vi "Device_Read.vi"(9 "queue out":refnum<queue>, 10 "Selected Count":i32, 11 "Device Handler pointer":i64[](array[numeric])) -> ()   [LabVIEW 2026]
uses:
  <vilib>/Platform/TimedLoop/XDataNode/timing_clust.ctl
  <vilib>/Platform/TimedLoop/XDataNode/nitl_modes.ctl
  <vilib>/Platform/TimedLoop/XDataNode/wakeup.ctl
  <vilib>/platform/TimedLoop/XDataNode/XDataNode.xnode
  <vilib>/Platform/TimedLoop/XDataNode/XDNodeRunTimeDep.lvlib
panel:
  in  "dataextraction":bool
  out "timed out? 3":bool
  out "concatenated string":string
  out "# elements in queue":i32
  out "element":u8[](array[numeric])
  out "timed out? 2":bool
  out "RX Return Value  2":i32
  out "CAN_Frame":u8[](array[numeric])
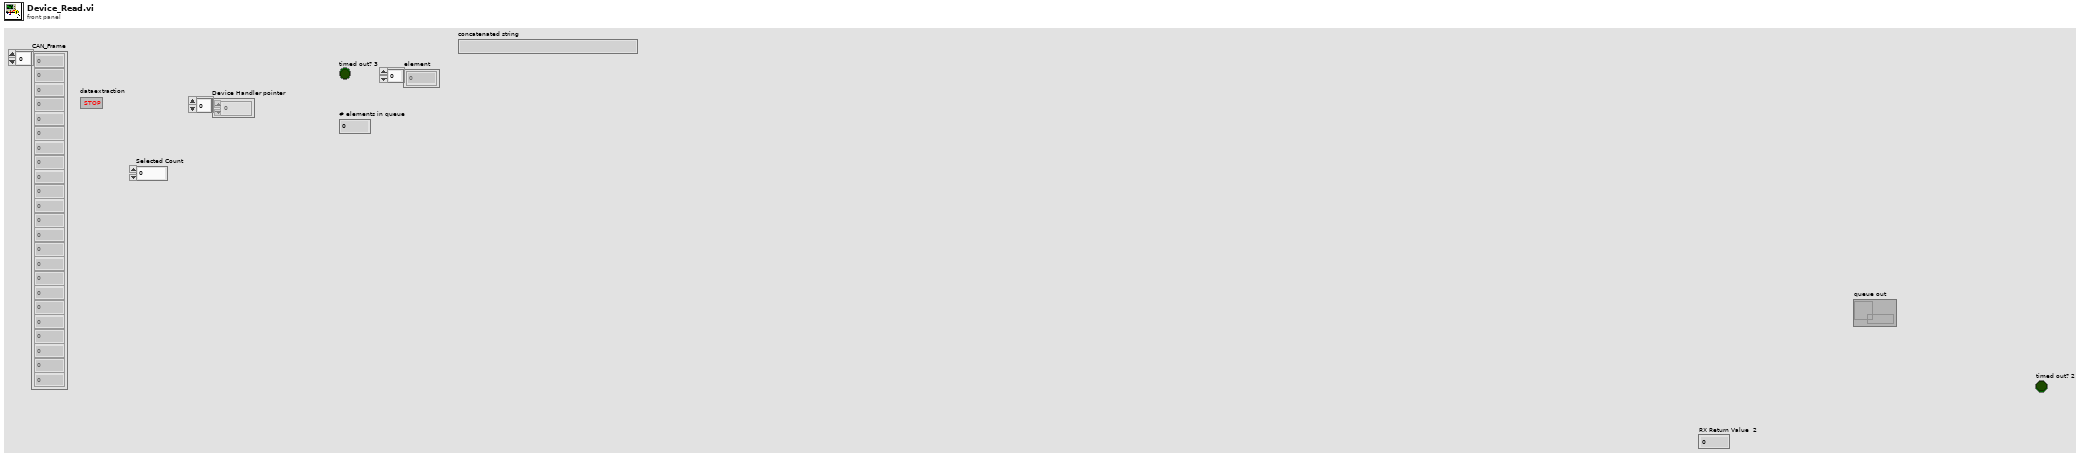
[diagram p1: front panel]
types:
  T1 = typedef "XDNodeRunTimeDep.lvlib/timing_clust.ctl" = cluster{"Expected End [f-1]":u64, "Actual End [f-1]":u64, "Finished Late? [f-1]":bool, "Expected End [i-1]":u64, "Actual End [i-1]":u64, "Finished Late? [i-1]":bool, "Expected Start [i]":u64, "Actual Start [i]":u64, "Expected Start [f]":u64, "Actual Start [f]":u64, "Source Name":string, "Structure Name":string, "Period":i64, "Deadline":i64, "Offset":i64, "Start":i64, "Priority":i32, "Timeout":i32, "Mode":T2, "Wakeup Reason":T3, "Error":errorcluster, "Source Type":string, "Secondary Source Type":string, "Global End Time":u64, "Global Start Time":u64, "Frame Duration":u64, "Iteration Duration":u64, "Assigned CPU":i32, "I/O Scan Engine Mode":u32}
  T2 = typedef "XDNodeRunTimeDep.lvlib/nitl_modes.ctl" = enum32{"No Change", "Process missed periods, maintain original phase", "Discard missed periods, maintain original phase", "Process missed periods, ignore original phase", "Discard missed periods, ignore original phase"}
  T3 = typedef "XDNodeRunTimeDep.lvlib/wakeup.ctl" = enum32{"Normal", "Aborted", "Asynchronous wakeup", "Timing source error", "Timed loop error", "Timeout"}
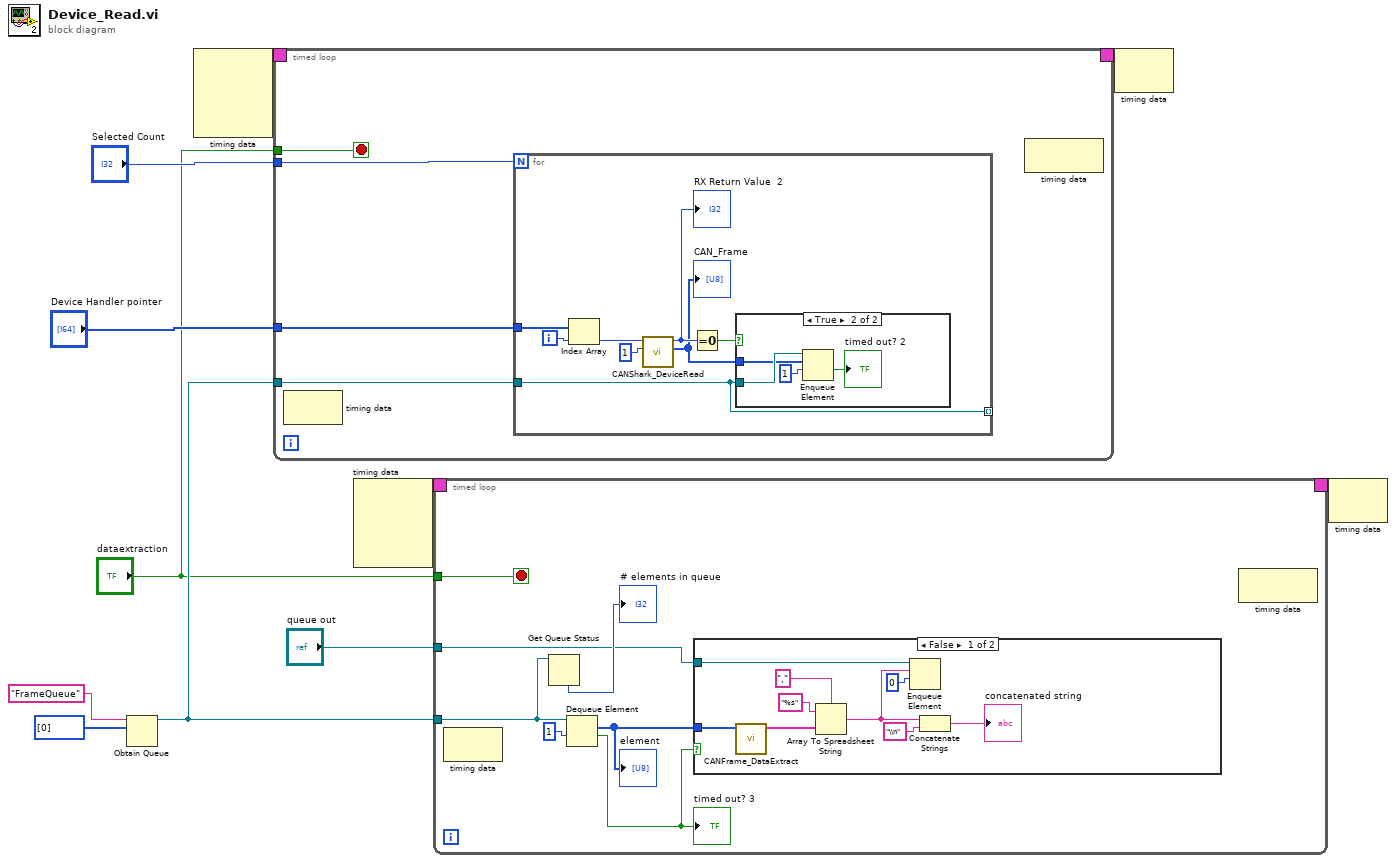
[diagram p0: block diagram]
diagram:
  n1 = Obtain Queue(name (unnamed)="FrameQueue", element data type=u8[] [0]) -> (queue out=w3:refnum<queue>)  [unwired: 3 in, 2 out]
  n2 = node-c288() -> (w11:T1)  [unwired: 4 in]
  n3 = timed-loop {
    timing: w11 -> [_]
    timing-out: [_] -> w10
    tunnel: "Device Handler pointer" -> [w15]
    tunnel: w3 -> [w14]
    tunnel: "Selected Count" -> [w13]
    tunnel: "dataextraction" -> [w12]
    stop <- w12 stop-if-true
    n4 = node-c288() -> ()  [unwired: 1 in, 1 out]
    n5 = for {
      N: w13 -> [_]
      tunnel: w15 -> [w21]
      tunnel: [w20] -> _ mode=indexing
      tunnel: w14 -> [w20]
      i -> [w22]
      n6 = Index Array(array=w21, index=w22) -> (element=w19:i64)
      n7 = call "CANShark_DeviceRead.vi"("Timeout"=1, "Device Handler"=w19) -> ("CAN_Frame"=w16:u8[], "RX Return Value"=w17:i32)  [unwired: 8 in]
      "RX Return Value  2" <- w17
      "CAN_Frame" <- w16
      n8 = Equal To 0?(x=w17) -> (x = 0?=w23:bool)
      n9 = case shown="True" w23 {
        tunnel: w20 -> [_ w26]
        tunnel: w16 -> [_ w24]
        frame False {
        }
        frame True {
          n10 = Enqueue Element(queue=w26, element=w24, timeout in ms (-1)=1) -> (timed out?=→"timed out? 2":bool)  [unwired: 1 in, 2 out]
        }
      }
    }
    n11 = node-c288() -> ()  [unwired: 1 in, 1 out]
  }
  n12 = node-c288() -> (w5:T1)  [unwired: 4 in]
  n13 = timed-loop {
    timing: w5 -> [_]
    timing-out: [_] -> w4
    tunnel: w3 -> [w32]
    tunnel: "dataextraction" -> [w31]
    tunnel: "queue out" -> [w30]
    stop <- w31 stop-if-true
    n14 = node-c288() -> ()  [unwired: 1 in, 1 out]
    n15 = Get Queue Status(queue=w32) -> (# elements in queue=→"# elements in queue":i32)  [unwired: 2 in, 7 out]
    n16 = Dequeue Element(queue=w32, timeout in ms (-1)=1) -> (element=w34:u8[], timed out?=w35:bool)  [unwired: 1 in, 2 out]
    "timed out? 3" <- w35
    "element" <- w34
    n17 = case shown="False" w35 {
      tunnel: w34 -> [w38 _]
      tunnel: w30 -> [w42 _]
      frame False {
        n18 = call "CANFrame_DataExtract.vi"("CANDATA"=w38) -> ("Extracted Data"=w37:string[])  [unwired: 10 in]
        n19 = Array To Spreadsheet String(delimiter (Tab)=",", array=w37, 3:"%s" ("format string")) -> (spreadsheet string=w40:string)
        n20 = Enqueue Element(queue=w42, element=w40, timeout in ms (-1)=0) -> ()  [unwired: 1 in, 3 out]
        n21 = Concatenate Strings(w40, "\\n" ("string")) -> (→"concatenated string":string)
      }
      frame True {
      }
    }
    n22 = node-c288() -> ()  [unwired: 1 in, 1 out]
  }
  n23 = node-c288(w10) -> ()  [unwired: 1 out]
  n24 = node-c288(w4) -> ()  [unwired: 1 out]
